vi "Load Transactions by Date.vi"(8 "error in (no error)":errorcluster, 10 "Year-Mo":string, 11 "Database in":refnum<class "Database.lvclass">) -> (0 "error out":errorcluster, 1 "Credit Statement":refnum<class "Statement.lvclass">, 2 "Bank Statement":refnum<class "Statement.lvclass">, 3 "Database out":refnum<class "Database.lvclass">)   [LabVIEW 2018, in "Database.lvclass"]
uses:
  Database.lvclass
  Statement/Statement.lvclass
  Banking Statement/Banking Statement.lvclass
  C:/Users/jtipps/Documents/Filthy-Lucre-Budgetizer/source/support/classes/Statement/Statement.lvclass
  Credit Statement/Credit Statement.lvclass
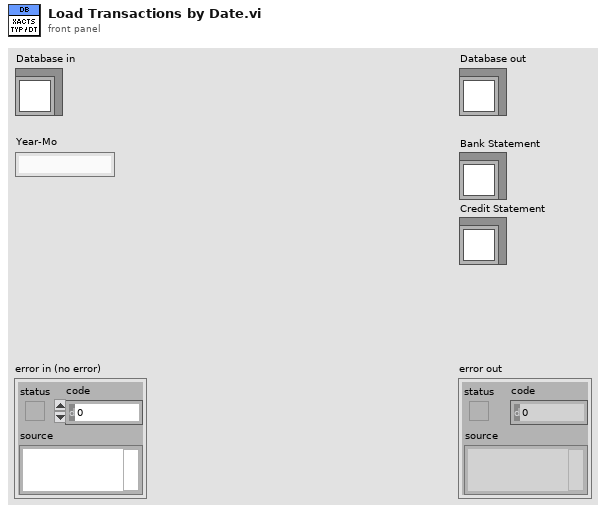
[diagram p1: front panel]
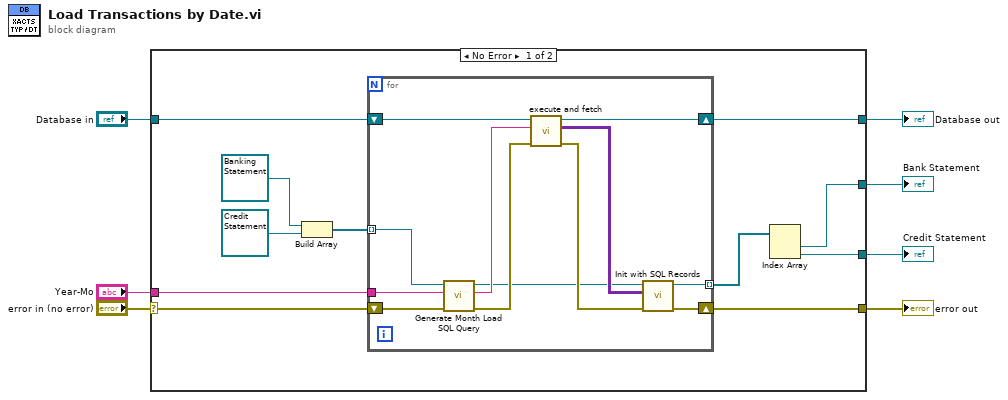
[diagram p0: block diagram]
diagram:
  n1 = case shown="No Error" "error in (no error)" {
    selector: "error in (no error)" -> [w15 w32]
    tunnel: [w16 w32] -> w6
    tunnel: [w17 w31] -> w4
    tunnel: "Database in" -> [w18 w31]
    tunnel: "Year-Mo" -> [w14 _]
    tunnel: [w9 _] -> w2
    tunnel: [w8 _] -> w1
    frame No Error {
      n2 = Build Array(refnum<class "Banking Statement.lvclass"> refnum ("Banking Statement.lvclass"), refnum<class "Credit Statement.lvclass"> refnum ("Credit Statement.lvclass")) -> (w11:refnum<class "Statement.lvclass">[])
      n3 = for {
        tunnel: w14 -> [w22]
        shift-right: [w25] -> w17
        shift-left: w18 -> [w26]
        shift-right: [w24] -> w16
        shift-left: w15 -> [w23]
        tunnel: w11 -> [w21] mode=indexing
        tunnel: [w19] -> w10 mode=indexing
        n4 = call-dynamic "Generate Month Load SQL Query.vi"("error in (no error)"=w23, "Year-Mo"=w22, "Statement in"=w21) -> ("error out"=w28:errorcluster, "SQL Query"=w29:string, "Statement out"=w20:refnum<class "Statement.lvclass">)  [unwired: 6 in]
        n5 = call "execute and fetch.vi"("error in (no error)"=w28, "SQL query"=w29, "Database in"=w26) -> ("error out"=w27:errorcluster, "recordset data"=w30:variant[][], "Database out"=w25:refnum<class "Database.lvclass">)  [unwired: 5 in, 1 out]
        n6 = call-dynamic "Init with SQL Records.vi"("error in (no error)"=w27, "SQL Dataset"=w30, "Statement in"=w20) -> ("error out"=w24:errorcluster, "Statement out"=w19:refnum<class "Statement.lvclass">)  [unwired: 7 in]
      }
      n7 = Index Array(array=w10) -> (element #1=w9:refnum<class "Statement.lvclass">, element #2=w8:refnum<class "Statement.lvclass">)  [unwired: 2 in]
    }
    frame Error {
    }
  }
  "error out" <- w6
  "Database out" <- w4
  "Bank Statement" <- w2
  "Credit Statement" <- w1
